vi "Get All Methods from LVClass Path.vi"(8 "error in":errorcluster, 10 "class path":path) -> (0 "error out":errorcluster, 2 "Methods":path[](array[path]))   [LabVIEW 2011, in "VITesterUtilities.lvlib"]
uses:
  Libraries/VITesterUtilities.lvlib
  <userlib>/_OpenG.lib/array/array.llb/Conditional Auto-Indexing Tunnel (String)__ogtk.vi
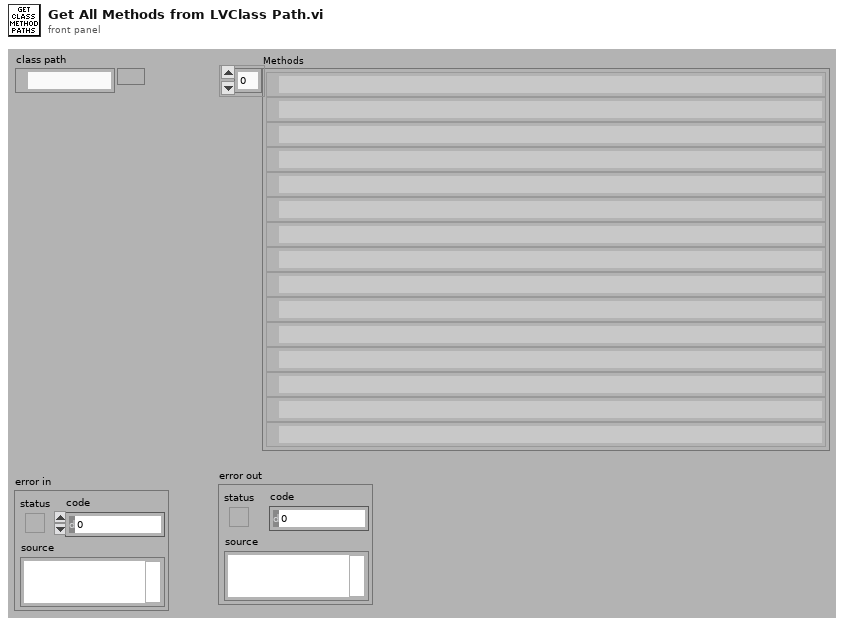
[diagram p1: front panel]
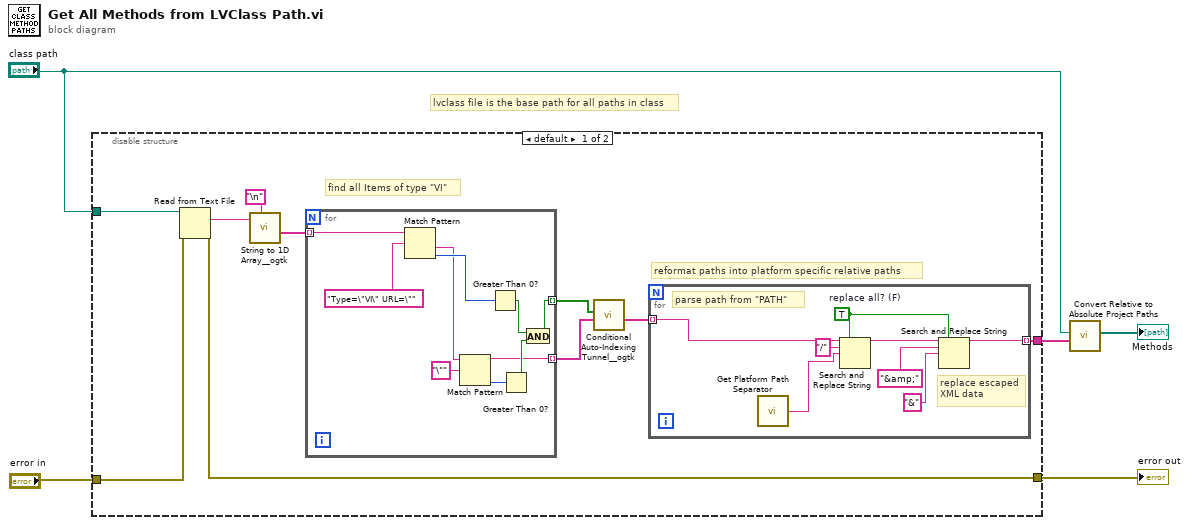
[diagram p0: block diagram]
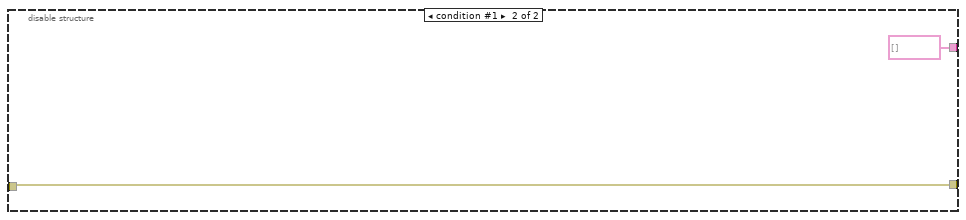
[diagram p2: hidden frame]
diagram:
  # "lvclass file is the base path for all paths in class"
  n1 = disable-structure shown="default" {
    disable-tunnel: "error in" -> [w15 w34]
    disable-tunnel: [w14 w34] -> w4
    disable-tunnel: [w13 string[] []] -> w3
    disable-tunnel: "class path" -> [w12 _]
    frame condition #0 (active) {
      # "find all Items of type \"VI\""
      # "reformat paths into platform specific relative paths"
      n2 = Read from Text File(file (use dialog)=w12, error in=w15) -> (text=w10:string, error out=w14:errorcluster)  [unwired: 2 in, 2 out]
      n3 = call <userlib>:"String to 1D Array__ogtk.vi"("delimiter (Tab)"="\n", "string"=w10) -> ("Array of Strings"=w7:string[])  [unwired: 9 in]
      n4 = for {
        tunnel: w7 -> [w33] mode=indexing
        tunnel: [w25] -> w8 mode=indexing
        tunnel: [w24] -> w11 mode=indexing
        n5 = Match Pattern(string=w33, regular expression="Type=\"VI\" URL=\"") -> (after substring=w30:string, offset past match=w31:i32)  [unwired: 1 in, 2 out]
        n6 = Match Pattern(string=w30, regular expression="\"") -> (before substring=w24:string, offset past match=w28:i32)  [unwired: 1 in, 2 out]
        n7 = Greater Than 0?(x=w31) -> (x > 0?=w26:bool)
        n8 = Greater Than 0?(x=w28) -> (x > 0?=w27:bool)
        n9 = And(x=w26, y=w27) -> (x .and. y?=w25:bool)
      }
      n10 = call-poly <userlib>:"Conditional Auto-Indexing Tunnel__ogtk.vi"("Array in"=w11, "Elements to keep"=w8) -> ("Filtered Array out"=w9:string[])  [unwired: 5 in]
      n11 = for {
        tunnel: w9 -> [w21] mode=indexing
        tunnel: [w17] -> w13 mode=indexing
        w16 = TRUE  # replace all? (F)
        # "replace escaped\nXML data"
        # "parse path from \"PATH\""
        n12 = call "Get Platform Path Separator.vi"() -> ("platform path separator"=w22:string)
        n13 = Search and Replace String(replace all?=w16, input string=w21, search string="/", replace string=w22) -> (result string=w20:string)  [unwired: 4 in, 3 out]
        n14 = Search and Replace String(replace all?=w16, input string=w20, search string="&amp;" ("replace string (\"\")"), replace string="&" ("replace string (\"\")")) -> (result string=w17:string)  [unwired: 4 in, 3 out]
      }
    }
    frame condition #1 {
    }
  }
  "error out" <- w4
  n15 = call "Convert Relative to Absolute Project Paths.vi"("VI Relative Paths"=w3, "Project File"="class path") -> ("VI Absolute Paths"=→"Methods":path[])  [unwired: 9 in]
